vi "AH_READ.VI"(0 "AH2500A address":string="20") -> (1 "capacitance":dbl=nan format="%.8f", 2 "loss":dbl=nan format="%.8f")   [LabVIEW 2020]
panel:
  out "Vexc":dbl=nan format="%.8f"
  out "out string":string
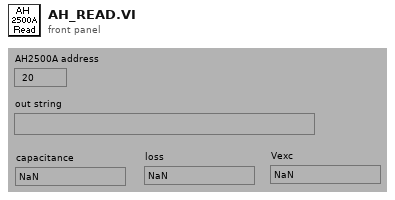
[diagram p1: front panel]
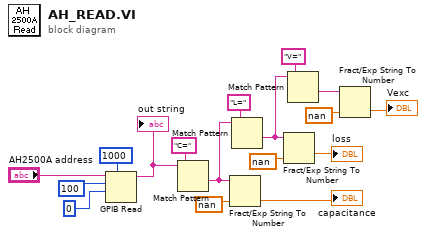
[diagram p0: block diagram]
diagram:
  n1 = GPIB Read(0:"AH2500A address", 1:100, 2:i16 0, 4:1000 ("timeout ms (488.2 global)")) -> (5:w12:string)  [unwired: 1 in, 2 out]
  "out string" <- w12
  n2 = Match Pattern(string=w12, regular expression="C=") -> (after substring=w7:string)  [unwired: 1 in, 3 out]
  n3 = Fract/Exp String To Number(string=w7, default (0 dbl)=nan) -> (number=→"capacitance":dbl)  [unwired: 2 in, 1 out]
  n4 = Match Pattern(string=w7, regular expression="L=") -> (after substring=w2:string)  [unwired: 1 in, 3 out]
  n5 = Fract/Exp String To Number(string=w2, default (0 dbl)=nan) -> (number=→"loss":dbl)  [unwired: 2 in, 1 out]
  n6 = Match Pattern(string=w2, regular expression="V=") -> (after substring=w5:string)  [unwired: 1 in, 3 out]
  n7 = Fract/Exp String To Number(string=w5, default (0 dbl)=nan) -> (number=→"Vexc":dbl)  [unwired: 2 in, 1 out]
